vi "显示位数写入.vi"(4 "error in (no error)":errorcluster caption="错误输入（无错误）", 5 "Value":u8 caption="值", 6 "Container State":T2 caption="容器状态", 7 "Display State In":T1={"显示位数"=6, "小数位数"=0} caption="显示状态输入") -> (0 "error out":errorcluster caption="错误输出", 3 "Display State Out":T1={"显示位数"=6, "小数位数"=0} caption="显示状态输出")   [LabVIEW 2013, in "数码管.xctl"]
uses:
  <vilib>/_xctls/Container State.ctl
  <vilib>/_xctls/XControlSupport.lvlib
panel:
  # "将以下值显示控件替换为所需类型的显示控件。\n不要从连线板中删除该显示控件或其它显示控件。\n不要更改连线板模式。\n值显示控件应始终位于连线板输出端自顶部起第三个接线端。"
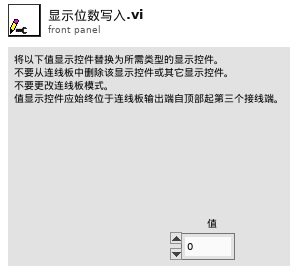
[diagram p1: front panel]
types:
  T1 = typedef "数码管.xctl/数码管.ctl" = cluster{"显示位数":u8, "小数位数":u8}
  T2 = typedef "XControlSupport.lvlib/Container State.ctl" = cluster{"Indicator?":bool, "Run Mode?":bool, " Refnum":refnum<vi>}
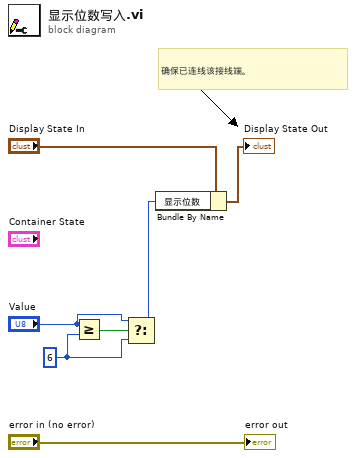
[diagram p0: block diagram]
diagram:
  w3 = u8 6 ("y")
  # "确保已连线该接线端。"
  n1 = Greater Or Equal?(x="Value", y=w3) -> (x >= y?=w4:bool)
  n2 = Select(t="Value", s=w4, f=w3) -> (s? t:f=w1:u8)
  n3 = Bundle By Name(cluster="Display State In", "显示位数"=w1) -> (→"Display State Out":T1)
  "error out" <- "error in (no error)"
